vi "Pert_Fdesired.vi"(0 "Time":dbl, 2 "Pert Param":dbl[](array[numeric])) -> (5 "condition":bool, 6 "y_Fdesired":dbl)   [LabVIEW 2017]
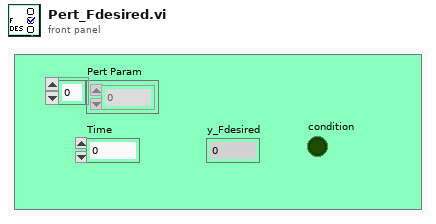
[diagram p1: front panel]
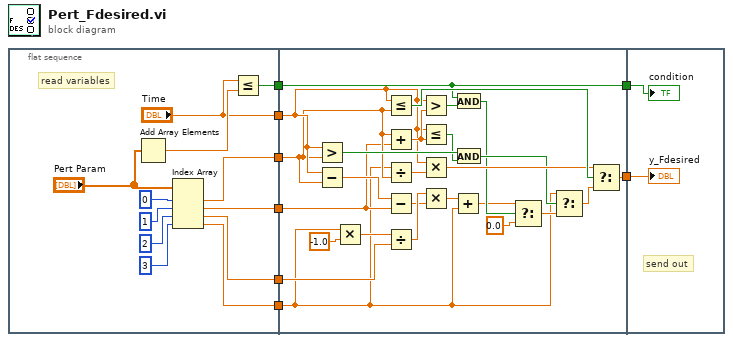
[diagram p0: block diagram]
diagram:
  n1 = flat-sequence {
    tunnel: [w16] -> w8
    tunnel: [w15] -> w7
    tunnel: [w14] -> w6
    tunnel: [w13] -> w5
    tunnel: [w11] -> w4
    tunnel: ["Time"] -> w2
    tunnel: w8 -> [w31]
    tunnel: w7 -> [w29]
    tunnel: w6 -> [w35]
    tunnel: w5 -> [w25]
    tunnel: w4 -> [w38]
    tunnel: [w38] -> w3
    tunnel: w2 -> [w32]
    tunnel: [w21] -> w1
    tunnel: w3 -> [w48]
    tunnel: w1 -> [w47]
    frame #0 {
      # "read variables"
      n2 = Add Array Elements(numeric array="Pert Param") -> (sum=w12:dbl)
      n3 = Index Array(array="Pert Param", index #1=0 ("index"), index #2=1 ("index"), index #3=2 ("index"), index #4=3 ("index")) -> (element #1=w16:dbl, element #2=w15:dbl, element #3=w14:dbl, element #4=w13:dbl)
      n4 = Less Or Equal?(x="Time", y=w12) -> (x <= y?=w11:bool)
    }
    frame #1 {
      n5 = Greater?(x=w32, y=w31) -> (0:w43:bool)
      n6 = Subtract(x=w32, y=w31) -> (x-y=w30:dbl)
      n7 = Multiply(x=w25, y=-1.0) -> (x*y=w34:dbl)
      n8 = Less Or Equal?(x=w32, y=w31) -> (x <= y?=w46:bool)
      n9 = Add(x=w31, y=w29) -> (x+y=w37:dbl)
      n10 = Divide(x=w25, y=w31) -> (x/y=w45:dbl)
      n11 = Subtract(x=w30, y=w29) -> (x-y=w27:dbl)
      n12 = Divide(x=w34, y=w35) -> (x/y=w28:dbl)
      n13 = Greater?(x=w32, y=w37) -> (0:w36:bool)
      n14 = Less Or Equal?(x=w32, y=w37) -> (x <= y?=w42:bool)
      n15 = Multiply(x=w32, y=w45) -> (x*y=w44:dbl)
      n16 = Multiply(x=w28, y=w27) -> (x*y=w26:dbl)
      n17 = Add(x=w26, y=w25) -> (x+y=w24:dbl)
      n18 = And(x=w38, y=w36) -> (x .and. y?=w39:bool)
      n19 = And(x=w43, y=w42) -> (x .and. y?=w41:bool)
      n20 = Select(t=w24, s=w39, f=0.0) -> (s? t:f=w40:dbl)
      n21 = Select(t=w25, s=w41, f=w40) -> (s? t:f=w23:dbl)
      n22 = Select(t=w44, s=w46, f=w23) -> (s? t:f=w21:dbl)
    }
    frame #2 {
      # "send out"
      "condition" <- w48
      "y_Fdesired" <- w47
    }
  }
